vi "Feedback Picture.vi"(5 "Unused":bool, 7 "Open State":T3, 10 "Closed State":T3, 11 "Feedback Pictures":T2) -> (2 "Feedback Picture":T1)   [LabVIEW 2020, in "VolatusGUI.lvlib" / "2WayValve.lvclass"]
uses:
  2WayValve.lvclass
  Channel State.ctl
  Feedback Pictures.ctl
  Picture.ctl
  2WayValve.lvclass/2WayValve.ctl
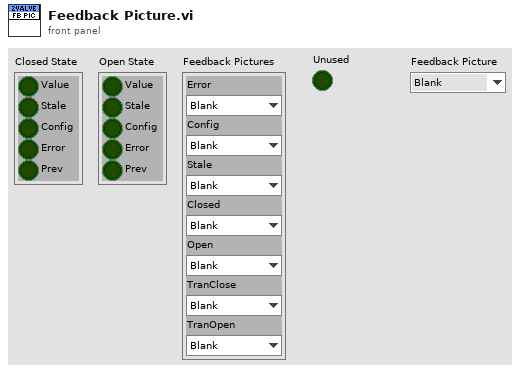
[diagram p1: front panel]
types:
  T1 = typedef "VolatusGUI.lvlib/2WayValve.lvclass/Picture.ctl" = enum16{"Blank", "OutClose", "OutOpen", "OutTranClose", "OutTranOpen", "OutConfig", "OutStale", "OutError", "InClose", "InOpen", "InTranClose", "InTranOpen", "InConfig", "InStale", "InError", "EnOff", "EnOn", "EnConfig", "EnStale", "EnError"}
  T2 = typedef "VolatusGUI.lvlib/2WayValve.lvclass/Feedback Pictures.ctl" = cluster{"Error":T1, "Config":T1, "Stale":T1, "Closed":T1, "Open":T1, "TranClose":T1, "TranOpen":T1}
  T3 = typedef "VolatusGUI.lvlib/2WayValve.lvclass/Channel State.ctl" = cluster{"Value":bool, "Stale":bool, "Config":bool, "Error":bool, "Prev":bool}
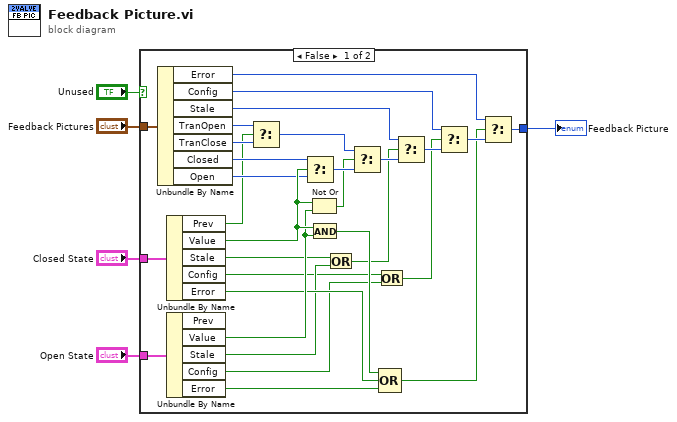
[diagram p0: block diagram]
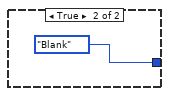
[diagram p2: hidden frame]
diagram:
  n1 = case shown="False" "Unused" {
    tunnel: "Feedback Pictures" -> [w35 _]
    tunnel: "Closed State" -> [w34 _]
    tunnel: "Open State" -> [w33 _]
    tunnel: [w12 Picture."Blank" ("Open")] -> w2
    frame False {
      n2 = Unbundle By Name(w35) -> ("Error"=w14:T1, "Config"=w19:T1, "Stale"=w21:T1, "TranOpen"=w11:T1, "TranClose"=w10:T1, "Closed"=w9:T1, "Open"=w8:T1)
      n3 = Unbundle By Name(w34) -> ("Prev"=w7:bool, "Value"=w30:bool, "Stale"=w24:bool, "Config"=w18:bool, "Error"=w27:bool)
      n4 = Unbundle By Name(w33) -> ("Value"=w29:bool, "Stale"=w23:bool, "Config"=w17:bool, "Error"=w28:bool)  [unwired: 1 out]
      n5 = Select(t=w11, s=w7, f=w10) -> (s? t:f=w6:T1)
      n6 = Select(t=w9, s=w30, f=w8) -> (s? t:f=w32:T1)
      n7 = Not Or(1:w29, 2:w30) -> (0:w31:bool)
      n8 = And(x=w30, y=w29) -> (x .and. y?=w26:bool)
      n9 = Or(x=w24, y=w23) -> (x .or. y?=w22:bool)
      n10 = Select(t=w6, s=w31, f=w32) -> (s? t:f=w25:T1)
      n11 = Or(x=w18, y=w17) -> (x .or. y?=w16:bool)
      n12 = Compound Arithmetic op=OR(w26, w27, w28) -> (w13:bool)
      n13 = Select(t=w21, s=w22, f=w25) -> (s? t:f=w20:T1)
      n14 = Select(t=w19, s=w16, f=w20) -> (s? t:f=w15:T1)
      n15 = Select(t=w14, s=w13, f=w15) -> (s? t:f=w12:T1)
    }
    frame True {
    }
  }
  "Feedback Picture" <- w2
